vi "TemperatureSensorSubVI.vi"(1 "Raw Input (V)":dbl, 2 "Offset (V)":dbl, 3 "Slope (V/C)":dbl) -> (0 "Temperature (C)":dbl)   [LabVIEW 2016]
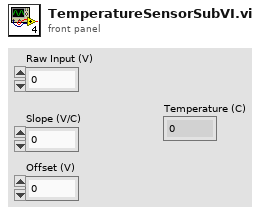
[diagram p1: front panel]
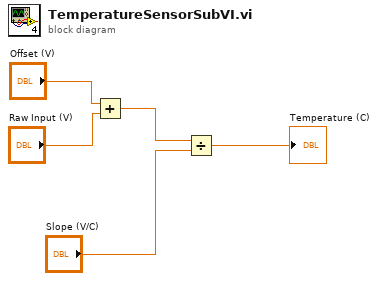
[diagram p0: block diagram]
diagram:
  n1 = Add(x="Offset (V)", y="Raw Input (V)") -> (x+y=w2:dbl)
  n2 = Divide(x=w2, y="Slope (V/C)") -> (x/y=→"Temperature (C)":dbl)
